vi "SimSharpness.vi"(1 "Focus Parameters":T1={"Z0"=3.0, "f0"=100.0, "curvature"=3.0, "noise"=2.0}, 2 "Z":dbl) -> (0 "Sharpness":dbl)   [LabVIEW 2014]
uses:
  <vilib>/express/express arith-compare/Formula/XNode/ExpressFormulaBlockNode.xnode
panel:
  # "LICENSED MATERIALS – PROPERTY OF IBM\nCopyright IBM Corp. 2016,\nALL RIGHTS RESERVED"
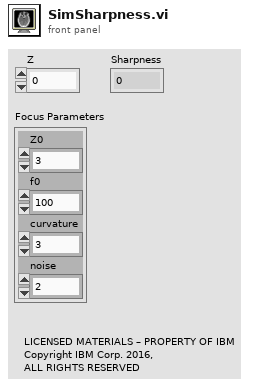
[diagram p1: front panel]
types:
  T1 = cluster{"Z0":dbl, "f0":dbl, "curvature":dbl, "noise":dbl}
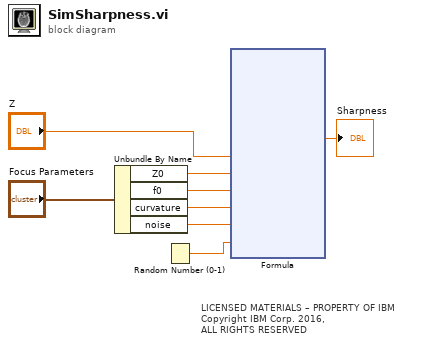
[diagram p0: block diagram]
diagram:
  # "LICENSED MATERIALS – PROPERTY OF IBM\nCopyright IBM Corp. 2016,\nALL RIGHTS RESERVED"
  n1 = Unbundle By Name("Focus Parameters") -> ("Z0"=w5:dbl, "f0"=w4:dbl, "curvature"=w3:dbl, "noise"=w2:dbl)
  n2 = Random Number (0-1)() -> (number: 0 to 1=w1:dbl)
  n3 = xnode "Formula"("Z"="Z", "Z0"=w5, "f0"=w4, "curvature"=w3, "noise"=w2, "rnd"=w1) -> ("Result"=→"Sharpness":dbl)  [unwired: 1 in, 1 out]
